vi "Virtual particle trace (forward).vi"(6 "U_inf":sgl[](array[numeric])=[1.0, 0.0, 0.0], 8 "r_max":sgl=10.0, 9 "dt":sgl=0.01, 10 "P_start":sgl[](array[numeric])=[0.0, 0.0, 0.0], 11 "Panel triangles in":T1[](array[typedef])) -> (0 "W":sgl[](array[numeric]), 1 "V":sgl[](array[numeric]), 2 "U":sgl[](array[numeric]), 3 "r":sgl[](array[numeric]), 4 "Completed":bool, 5 "Points":sgl[][](array[numeric]))   [LabVIEW 2017]
uses:
  ctls/Triangle panel.ctl
panel:
  out "r / r_max":sgl
  out "Progress":sgl(slide)=3330.0 scale=0.0..3330.0
  out "loop number":i32
  in  "Stop":bool
  # "If progress bar stops advancing while loop number continues increasing, press stop to exit the loop."
  # "Lack of progress is caused by a particle getting \"stuck\"."
  # "PN 26/10/17"
  # "Vertices"
  # "Edges"
  # "Unit normal"
  # "Control point"
  # "Edge\nlinks \n(tri index)"
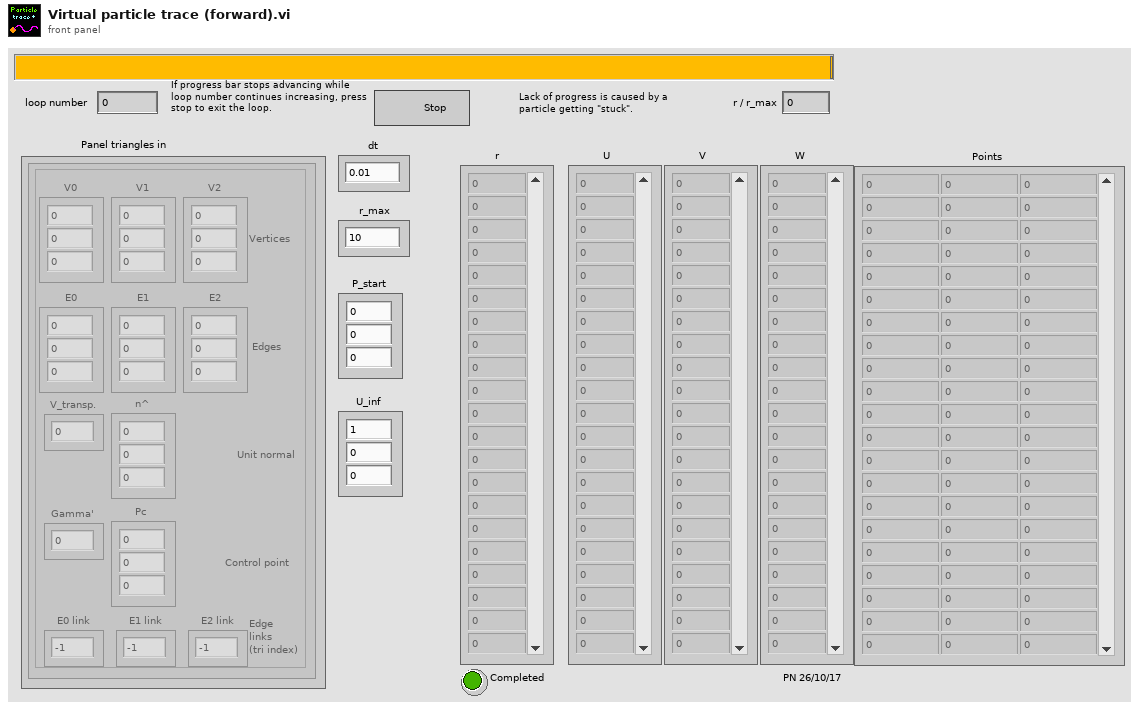
[diagram p1: front panel]
types:
  T1 = typedef "Triangle panel.ctl" = cluster{"V0":sgl[], "V1":sgl[], "V2":sgl[], "E0":sgl[], "E1":sgl[], "E2":sgl[], "n^":sgl[], "Pc":sgl[], "Gamma'":sgl, "V_transp.":sgl, "E0 link":i32, "E1 link":i32, "E2 link":i32}
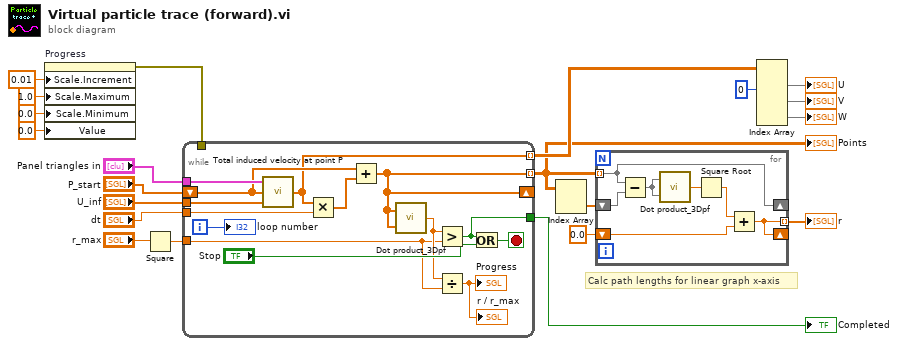
[diagram p0: block diagram]
diagram:
  # "Calc path lengths for linear graph x-axis"
  n1 = property on="Progress" class="Slide (strict)"("Scale.Increment"=0.01 ("Scale.Range:Increment"), "Scale.Maximum"=1.0 ("Scale.Range:Maximum"), "Scale.Minimum"=0.0 ("Scale.Range:Minimum"), "Value"=sgl 0.0 ("Progress")) -> (error out=w7:errorcluster)  [unwired: 2 in, 1 out]
  n2 = Square(x="r_max") -> (x^2=w12:sgl)
  n3 = while {
    tunnel: "U_inf" -> [w35]
    tunnel: "Panel triangles in" -> [w34]
    shift-right: [w26] -> _
    shift-left: "P_start" -> [w33]
    tunnel: "dt" -> [w32]
    tunnel: [w26] -> w1 mode=indexing
    tunnel: w12 -> [w24]
    tunnel: [w29] -> w16 mode=indexing
    tunnel: w7 -> [_]
    tunnel: [w22] -> w2
    i -> [w30]
    stop <- w28 stop-if-true
    n4 = call "Total induced velocity at point P.vi"("U_inf"=w35, "P"=w33, "Triangle panels"=w34) -> ("(U, V, W) at P"=w29:sgl[])
    n5 = Multiply(x=w29, y=w32) -> (x*y=w31:sgl[])
    n6 = Add(x=w33, y=w31) -> (x+y=w26:sgl[])
    n7 = call "Dot product_3Dpf.vi"("B"=w26, "A"=w26) -> ("A . B"=w25:sgl)
    n8 = Greater?(x=w25, y=w24) -> (0:w22:bool)
    n9 = Divide(x=w25, y=w24) -> (x/y=→"Progress" →"r / r_max":sgl)
    n10 = Or(x=w22, y="Stop") -> (x .or. y?=w28:bool)
    "loop number" <- w30
  }
  "Completed" <- w2
  "Points" <- w1
  n11 = Index Array(array=w1) -> (element=w18:sgl[])  [unwired: 2 in]
  n12 = for {
    tunnel: w1 -> [w38] mode=indexing
    shift-right: [w38] -> _
    shift-left: w18 -> [w42]
    tunnel: [w36] -> w3 mode=indexing
    shift-right: [w36] -> _
    shift-left: sgl 0.0 -> [w37]
    n13 = Subtract(x=w38, y=w42) -> (x-y=w41:sgl[])
    n14 = call "Dot product_3Dpf.vi"("B"=w41, "A"=w41) -> ("A . B"=w40:sgl)
    n15 = Square Root(x=w40) -> (sqrt(x)=w39:sgl)
    n16 = Add(x=w39, y=w37) -> (x+y=w36:sgl)
  }
  "r" <- w3
  n17 = Index Array(array=w16, index (col) #1=0 ("disabled index (col)")) -> (element #1=→"U":sgl[], element #2=→"V":sgl[], element #3=→"W":sgl[])  [unwired: 5 in]
